vi "VHRunnableVI.vi"(8 "error in (no error)":errorcluster, 10 "Paramters":string[](array[string])) -> (0 "error out":errorcluster)   [LabVIEW 2013, in "VIHost.lvlib"]
uses:
  VIHost.lvlib
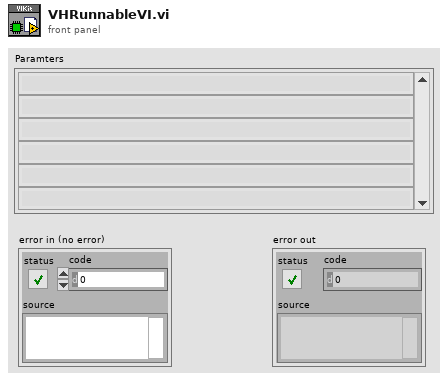
[diagram p1: front panel]
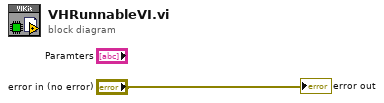
[diagram p0: block diagram]
diagram:
  "error out" <- "error in (no error)"
